vi "Create Message Queue_Sushu.vi"(0 "message queue name":string, 1 "max queue size (-1, unlimited)":i32=-1, 5 "initial message names":string, 7 "initial message values":string[](array[string]), 11 "error in":errorcluster) -> (4 "Queue":cluster{"Q":T1, "Name":string}, 15 "error out":errorcluster)   [LabVIEW 2021]
doc: "为了使用方便，对AMC进行的二次封装,输入多个命令时，直接在字符串内回车另起一行即可，有几行就有几个命名。20131229\nNon Reentrant。\n蒋松：jiangsong@outlook.com\n\nCreates a new local message queue or returns a reference to an existing message queue baseed on the queue name. You can pass in a list of initial messages which will be added to the queue."
uses:
  <vilib>/NI/AMC/Message Queue.ctl
  <vilib>/NI/AMC/Message.ctl
  <vilib>/NI/Tools/Keyed Array/KeyedArray.ctl
  <vilib>/NI/AMC/AMC.lvlib
  <vilib>/NI/Tools/Keyed Array/Tools_KeyedArray.lvlib
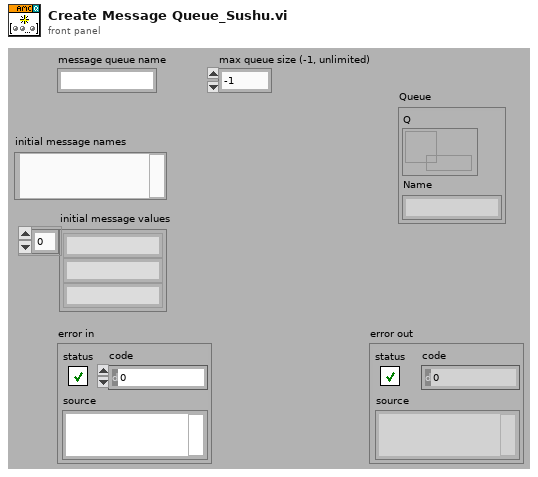
[diagram p1: front panel]
types:
  T1 = typedef "AMC.lvlib/Message Queue.ctl" = refnum<queue>
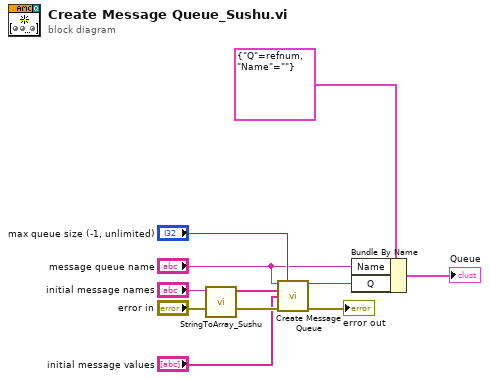
[diagram p0: block diagram]
diagram:
  n1 = call <userlib>:"StringToArray_Sushu.vi"("State Queue"="initial message names") -> ("Array"=w5:string[])  [unwired: 7 in, 3 out]
  n2 = call <vilib>:"Create Message Queue.vi"("message queue name"="message queue name", "max queue size (-1, unlimited)"="max queue size (-1, unlimited)", "initial message names"=w5, "initial message values"="initial message values", "error in"="error in") -> ("message queue out"=w3:T1, "error out"=→"error out":errorcluster)  [unwired: 9 in]
  n3 = Bundle By Name(cluster=cluster{"Q":T1, "Name":string} {"Q"=refnum, "Name"=""} ("Queue"), "Name"="message queue name", "Q"=w3) -> (→"Queue":cluster{"Q":T1, "Name":string})
